vi "Image acquisition polarization camera - polling.vi"() -> ()   [LabVIEW 2015]
uses:
  SubVIs/Parameters Get & Set/Get Parameters/Get NumberOfQueuedFrames.vi
  SubVIs/Parameters Get & Set/Set Parameters/Set Gain.vi
  SubVIs/Parameters Get & Set/Get Parameters/Get CameraSensorType.vi
  SubVIs/Parameters Get & Set/Set Parameters/Set ExposureTime_us.vi
  SubVIs/Parameters Get & Set/Set Parameters/Set FramesPerTrigger_zeroForUnlimited.vi
  SubVIs/Parameters Get & Set/Set Parameters/Set OperationMode.vi
  C:/code/Host/Installer/Scientific Camera Interfaces/LabVIEW/64_bit/Library_X64/Thorlabs.TSI.TLCameraInterfaces.dll
  64_bit/Library_X64/Thorlabs.TSI.TLCameraInterfaces.dll
  C:/code/Host/Installer/Scientific Camera Interfaces/LabVIEW/64_bit/Library_X64/Thorlabs.TSI.PolarizationProcessor.dll
  64_bit/Library_X64/Thorlabs.TSI.PolarizationProcessor.dll
  C:/code/Host/Installer/Scientific Camera Interfaces/LabVIEW/64_bit/Library_X64/Thorlabs.TSI.PolarizationInterfaces.dll
  64_bit/Library_X64/Thorlabs.TSI.PolarizationInterfaces.dll
  SubVIs/Parameters Get & Set/Get Parameters/Get ROIAndBin.vi
  SubVIs/Parameters Get & Set/Get Parameters/Get PolarPhase.vi
  Controls/Polarization Processing Type.ctl
panel:
  out "Intensity Graph":dbl[][](graph)
  in  "Polarization Processing Type":T1
  in  "stop":bool
  out "FrameNumber":u32
  in  "Exposure (ms)":u32=30
  in  "Gain":u32 max=1023
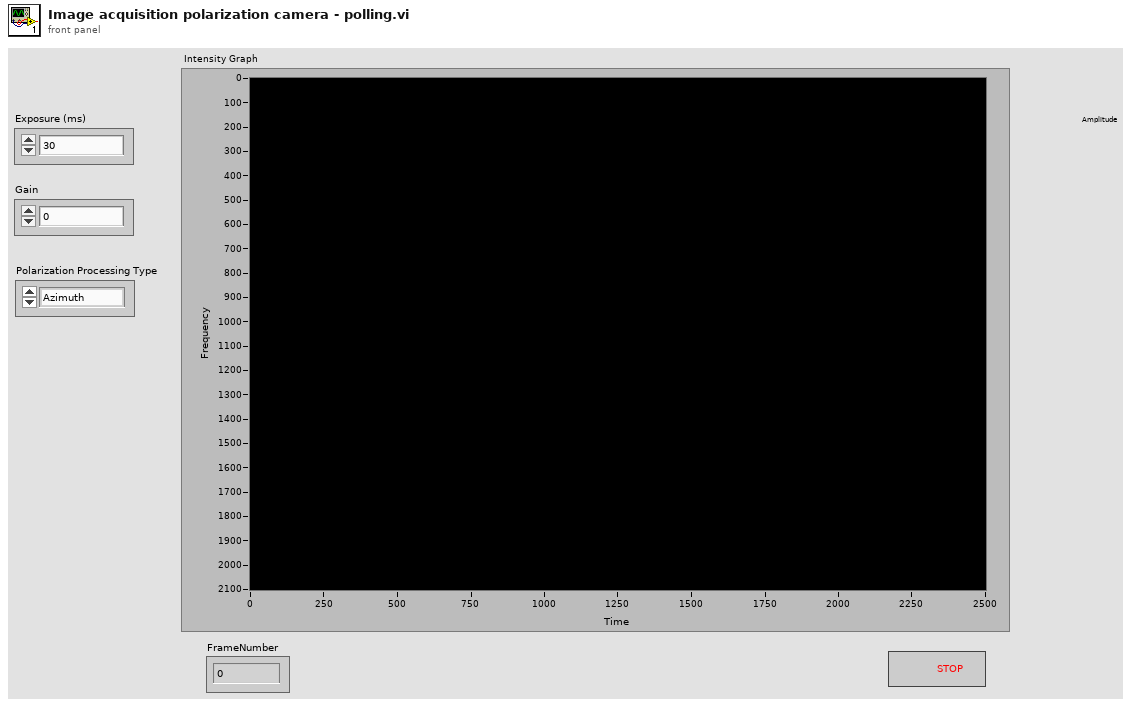
[diagram p1: front panel]
types:
  T1 = typedef "Polarization Processing Type.ctl" = enum16{"Azimuth", "DoLP", "Intensity"}
  T2 = enum8{"Enabled", "Disabled", "Disabled and Grayed Out"}
  T3 = typedef "Region of Interest.ctl" = cluster{"Origin - X":u32, "Origin - Y":u32, "Width":u32, "Height":u32}
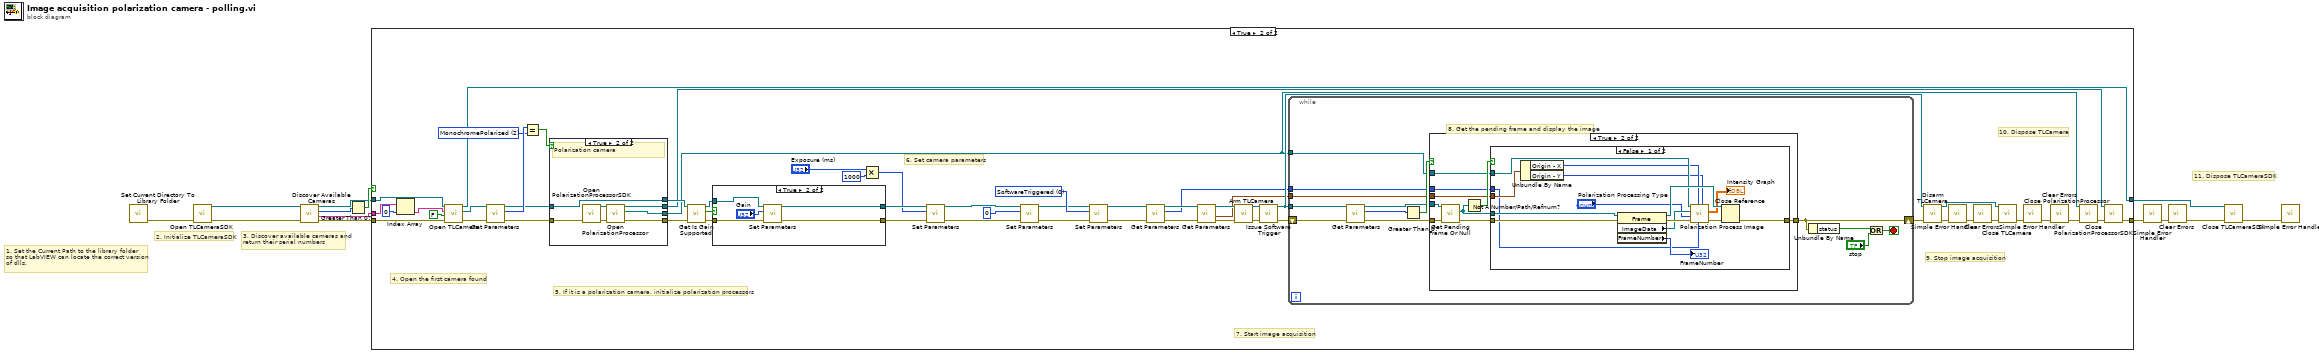
[diagram p0: block diagram]
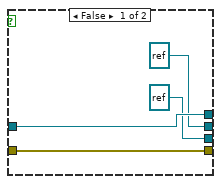
[diagram p3: hidden frame]
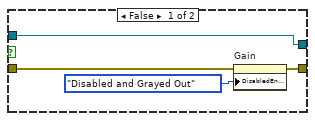
[diagram p4: hidden frame]
diagram:
  # "1. Set the Current Path to the library folder\nso that LabVIEW can locate the correct version\nof dlls."
  # "11. Dispose TLCameraSDK"
  # "3. Discover available cameras and\nreturn their serial numbers"
  # "2. Initialize TLCameraSDK"
  n1 = call "Set Current Directory To Library Folder.vi"() -> ("error out"=w7:errorcluster)  [unwired: 11 in]
  n2 = call "Open TLCameraSDK.vi"("error in (no error)"=w7) -> ("error out"=w6:errorcluster, "Thorlabs.TSI.TLCameraInterfaces.ITLCameraSDK"=w5:refnum<k24>)  [unwired: 9 in]
  n3 = call "Discover Available Cameras.vi"("error in (no error)"=w6, "Thorlabs.TSI.TLCameraInterfaces.ITLCameraSDK"=w5) -> ("error out"=w11:errorcluster, "Serial Numbers"=w8:string[], "Number of Cameras"=w10:i32, "Thorlabs.TSI.TLCameraInterfaces.ITLCameraSDK"=w9:refnum<k24>)  [unwired: 6 in]
  n4 = Greater Than 0?(x=w10) -> (x > 0?=w12:bool)
  n5 = case shown="True" w12 {
    tunnel: w9 -> [w14 w69]
    tunnel: w11 -> [w15 w55]
    tunnel: [w15 w26] -> w1
    tunnel: [w14 w66] -> w13
    tunnel: w8 -> [_ w64]
    frame False {
    }
    frame True {
      w34 = 2 items=["Monochrome", "Bayer", "MonochromePolarized"] ("CameraSensorType")
      w46 = 0 items=["SoftwareTriggered", "HardwareTriggered", "Bulb", "Reserved1", "Reserved2"] ("OperationMode")
      # "10. Dispose TLCamera"
      # "9. Stop image acquisition"
      # "7. Start image acquisition"
      # "6. Set camera parameters"
      # "5. If it is a polarization camera, initialize polarization processors"
      # "4. Open the first camera found"
      n6 = Index Array(array=w64, index=0) -> (element=w54:string)
      n7 = call "Open TLCamera.vi"("error in (no error)"=w55, "isDiagnosticsMessagesEnabled"=FALSE, "Camera serial number"=w54, "Thorlabs.TSI.TLCameraInterfaces.ITLCameraSDK"=w69) -> ("error out"=w52:errorcluster, "Thorlabs.TSI.TLCameraInterfaces.ITLCamera"=w53:refnum<k24>, "Thorlabs.TSI.TLCameraInterfaces.ITLCameraSDK"=w66:refnum<k24>)  [unwired: 5 in]
      n8 = call-poly "Get Parameters.vi"("error in (no error)"=w52, "Thorlabs.TSI.TLCameraInterfaces.ITLCamera"=w53) -> ("error out"=w31:errorcluster, "CameraSensorType"=w35:i32, "Thorlabs.TSI.TLCameraInterfaces.ITLCamera"=w32:refnum<k24>)  [unwired: 7 in]
      n9 = Equal?(x=w35, y=w34) -> (x = y?=w33:bool)
      n10 = case shown="True" w33 {
        tunnel: w32 -> [w73 w80]
        tunnel: w31 -> [w72 w79]
        tunnel: [w73 w80] -> w30
        tunnel: [w72 w76] -> w29
        tunnel: [refnum<k24> refnum ("PolarizationProcessorSDK reference out") w75] -> w25
        tunnel: [refnum<k24> refnum ("PolarizationProcessor reference") w74] -> w24
        frame False {
        }
        frame True {
          # "Polarization camera"
          n11 = call "Open PolarizationProcessorSDK.vi"("error in (no error)"=w79) -> ("error out"=w78:errorcluster, "Thorlabs.TSI.PolarizationProcessor.PolarizationProcessorSDK"=w77:refnum<k24>)  [unwired: 9 in]
          n12 = call "Open PolarizationProcessor.vi"("error in (no error)"=w78, "Thorlabs.TSI.PolarizationProcessor.PolarizationProcessorSDK"=w77) -> ("error out"=w76:errorcluster, "Thorlabs.TSI.PolarizationInterfaces.IPolarizationProcessor"=w74:refnum<k24>, "Thorlabs.TSI.PolarizationProcessor.PolarizationProcessorSDK"=w75:refnum<k24>)  [unwired: 7 in]
        }
      }
      n13 = call "Get Is Gain Supported.vi"("error in (no error)"=w29, "Thorlabs.TSI.TLCameraInterfaces.ITLCamera"=w30) -> ("error out"=w57:errorcluster, "Is Gain Supported?"=w59:bool, "Thorlabs.TSI.TLCameraInterfaces.ITLCamera"=w58:refnum<k24>)  [unwired: 7 in]
      n14 = case shown="True" w59 {
        tunnel: w58 -> [w81 w87]
        tunnel: w57 -> [w82 w89]
        tunnel: [w83 w88] -> w50
        tunnel: [w81 w86] -> w56
        frame False {
          n15 = property on="Gain" class="DigNum (strict)"(error in=w82, "DisabledEnum"=T2."Disabled and Grayed Out" ("Disabled")) -> (error out=w83:errorcluster)  [unwired: 1 in, 1 out]
        }
        frame True {
          n16 = call-poly "Set Parameters.vi"("error in (no error)"=w89, "Gain"="Gain", "Thorlabs.TSI.TLCameraInterfaces.ITLCamera"=w87) -> ("error out"=w88:errorcluster, "Thorlabs.TSI.TLCameraInterfaces.ITLCamera"=w86:refnum<k24>)  [unwired: 7 in]
        }
      }
      n17 = Multiply(x="Exposure (ms)", y=u32 1000) -> (x*y=w51:u32)
      n18 = call-poly "Set Parameters.vi"("error in (no error)"=w50, "ExposureTime_us"=w51, "Thorlabs.TSI.TLCameraInterfaces.ITLCamera"=w56) -> ("error out"=w47:errorcluster, "Thorlabs.TSI.TLCameraInterfaces.ITLCamera"=w48:refnum<k24>)  [unwired: 7 in]
      n19 = call-poly "Set Parameters.vi"("error in (no error)"=w47, "FramesPerTrigger_zeroForUnlimited"=u32 0 ("FramesPerTriggerOrZeroForUnlimited"), "Thorlabs.TSI.TLCameraInterfaces.ITLCamera"=w48) -> ("error out"=w44:errorcluster, "Thorlabs.TSI.TLCameraInterfaces.ITLCamera"=w45:refnum<k24>)  [unwired: 7 in]
      n20 = call-poly "Set Parameters.vi"("error in (no error)"=w44, "OperationMode"=w46, "Thorlabs.TSI.TLCameraInterfaces.ITLCamera"=w45) -> ("error out"=w20:errorcluster, "Thorlabs.TSI.TLCameraInterfaces.ITLCamera"=w18:refnum<k24>)  [unwired: 7 in]
      n21 = call-poly "Get Parameters.vi"("error in (no error)"=w20, "Thorlabs.TSI.TLCameraInterfaces.ITLCamera"=w18) -> ("error out"=w19:errorcluster, "PolarPhase"=w16:i32, "Thorlabs.TSI.TLCameraInterfaces.ITLCamera"=w17:refnum<k24>)  [unwired: 7 in]
      n22 = call-poly "Get Parameters.vi"("error in (no error)"=w19, "Thorlabs.TSI.TLCameraInterfaces.ITLCamera"=w17) -> ("error out"=w23:errorcluster, "Region of Interest"=w21:T3, "Thorlabs.TSI.TLCameraInterfaces.ITLCamera"=w22:refnum<k24>)  [unwired: 6 in, 1 out]
      n23 = call "Arm TLCamera.vi"("error in (no error)"=w23, "Thorlabs.TSI.TLCameraInterfaces.ITLCamera"=w22) -> ("error out"=w36:errorcluster, "Thorlabs.TSI.TLCameraInterfaces.ITLCamera"=w37:refnum<k24>)  [unwired: 8 in]
      n24 = call "Issue Software Trigger.vi"("error in (no error)"=w36, "Thorlabs.TSI.TLCameraInterfaces.ITLCamera"=w37) -> ("error out"=w62:errorcluster, "Thorlabs.TSI.TLCameraInterfaces.ITLCamera"=w63:refnum<k24>)  [unwired: 8 in]
      n25 = while {
        tunnel: w63 -> [w102]
        shift-right: [w99] -> w43
        shift-left: w62 -> [w95]
        tunnel: w24 -> [w92]
        tunnel: w21 -> [w91]
        tunnel: w16 -> [w90]
        stop <- w96 stop-if-true
        # "8. Get the pending frame and display the image"
        n26 = call-poly "Get Parameters.vi"("error in (no error)"=w95, "Thorlabs.TSI.TLCameraInterfaces.ITLCamera"=w102) -> ("error out"=w93:errorcluster, "NumberOfQueuedFrames"=w94:i32, "Thorlabs.TSI.TLCameraInterfaces.ITLCamera"=w100:refnum<k24>)  [unwired: 7 in]
        n27 = Greater Than 0?(x=w94) -> (x > 0?=w101:bool)
        n28 = case shown="True" w101 {
          tunnel: w93 -> [w103 w109]
          tunnel: w100 -> [_ w112]
          tunnel: [w103 w110] -> w99
          tunnel: w92 -> [_ w106]
          tunnel: w91 -> [_ w105]
          tunnel: w90 -> [_ w104]
          frame False {
          }
          frame True {
            n29 = call "Get Pending Frame Or Null.vi"("error in (no error)"=w109, "Thorlabs.TSI.TLCameraInterfaces.ITLCamera"=w112) -> ("error out"=w108:errorcluster, "Thorlabs.TSI.TLCameraInterfaces.Frame"=w107:refnum<k24>)  [unwired: 7 in, 1 out]
            n30 = Not A Number/Path/Refnum?(number/path/refnum=w107) -> (NaN/Path/Refnum?=w111:bool)
            n31 = case shown="False" w111 {
              tunnel: w107 -> [w127 _]
              tunnel: w108 -> [w126 w128]
              tunnel: [w124 w128] -> w110
              tunnel: w106 -> [w119 _]
              tunnel: w105 -> [w118 _]
              tunnel: w104 -> [w114 _]
              frame False {
                n32 = Unbundle By Name(w118) -> ("Origin - X"=w117:u32, "Origin - Y"=w116:u32)
                n33 = property class="Frame"(reference=w127, error in=w126) -> (reference out=w125:refnum<k24>, error out=w122:errorcluster, "ImageData"=w120:refnum<k24>, "FrameNumber"=→"FrameNumber":u32)
                n34 = call "Polarization Process Image.vi"("imageOriginY_pixels"=w116, "sensorPolarPhase"=w114, "imageOriginX_pixels"=w117, "error in (no error)"=w122, "Polarization Processing Type"="Polarization Processing Type", "Thorlabs.TSI.ImageDataInterfaces.IImageData"=w120, "Thorlabs.TSI.PolarizationInterfaces.IPolarizationProcessor"=w119) -> ("error out"=w121:errorcluster, "Output image data"=→"Intensity Graph":dbl[][])  [unwired: 2 in, 1 out]
                n35 = Close Reference(reference=w125, error in (no error)=w121) -> (error out=w124:errorcluster)
              }
              frame True {
              }
            }
          }
        }
        n36 = Unbundle By Name(w99) -> ("status"=w98:bool)
        n37 = Or(x=w98, y="stop") -> (x .or. y?=w96:bool)
      }
      n38 = call "Disarm TLCamera.vi"("error in (no error)"=w43, "Thorlabs.TSI.TLCameraInterfaces.ITLCamera"=w63) -> ("error out"=w42:errorcluster, "Thorlabs.TSI.TLCameraInterfaces.ITLCamera"=w67:refnum<k24>)  [unwired: 8 in]
      n39 = call <vilib>:"Simple Error Handler.vi"("error in (no error)"=w42) -> ("error out"=w41:errorcluster)  [unwired: 4 in, 4 out]
      n40 = call <vilib>:"Clear Errors.vi"("error in (no error)"=w41) -> ("error out"=w40:errorcluster)  [unwired: 5 in, 1 out]
      n41 = call "Close TLCamera.vi"("error in (no error)"=w40, "Thorlabs.TSI.TLCameraInterfaces.ITLCamera"=w67) -> ("error out"=w38:errorcluster)  [unwired: 9 in]
      n42 = call <vilib>:"Simple Error Handler.vi"("error in (no error)"=w38) -> ("error out"=w39:errorcluster)  [unwired: 4 in, 4 out]
      n43 = call <vilib>:"Clear Errors.vi"("error in (no error)"=w39) -> ("error out"=w28:errorcluster)  [unwired: 5 in, 1 out]
      n44 = call "Close PolarizationProcessor.vi"("error in (no error)"=w28, "Thorlabs.TSI.PolarizationInterfaces.IPolarizationProcessor"=w24) -> ("error out"=w27:errorcluster)  [unwired: 9 in]
      n45 = call "Close PolarizationProcessorSDK.vi"("error in (no error)"=w27, "Thorlabs.TSI.PolarizationProcessor.PolarizationProcessorSDK"=w25) -> ("error out"=w26:errorcluster)  [unwired: 9 in]
    }
  }
  n46 = call <vilib>:"Simple Error Handler.vi"("error in (no error)"=w1) -> ("error out"=w3:errorcluster)  [unwired: 4 in, 4 out]
  n47 = call <vilib>:"Clear Errors.vi"("error in (no error)"=w3) -> ("error out"=w2:errorcluster)  [unwired: 5 in, 1 out]
  n48 = call "Close TLCameraSDK.vi"("error in (no error)"=w2, "Thorlabs.TSI.TLCameraInterfaces.ITLCameraSDK"=w13) -> ("error out"=w4:errorcluster)  [unwired: 9 in]
  n49 = call <vilib>:"Simple Error Handler.vi"("error in (no error)"=w4) -> ()  [unwired: 4 in, 5 out]
